vi "Straighten Up V2015.vi"(2 "stop":bool, 3 "10CM?":bool, 4 "Estimated Location":u16(ring) items=["Center Top", "Left Top", "Center Bottom", "Right Bottom", "Home", "Right mid", "Center Top 0", "Panting rowe"]) -> (0 "X Guess":i32, 1 "Y Guess":i32)   [LabVIEW 2014]
uses:
  <vilib>/userdefined/High Color/nirio_resource_hc.ctl
  <vilib>/FPGAPlugInAG/myRIO-1900/niLvFpga_Open_myRIO-1900.vi
  <vilib>/rvi/interface/common/dynamic/niFpgaDynamicAddResources.vi
  <vilib>/Utility/error.llb/Error Cluster From Error Code.vi
  <vilib>/rvi/errors/niLvFpgaAdjustHostInterfaceError.vi
  <vilib>/FPGAPlugInAG/Dynamic/niLvFpga_Close_Dynamic.vi
  <vilib>/rvi/interface/nirviOpenFPGA/nirviOpenFPGA.xnode
  FPGA Bitfiles/MITe2015_FPGATarget_FPGA-1900MotorAu_fQqeE40Xepw.lvbitx
  FPGA/FPGA-1900 Motor Automation Test.vi
  <vilib>/rvi/interface/nirviReadWriteControl/nirviReadWriteControl.xnode
  <vilib>/rvi/interface/nirviCloseFPGA/nirviCloseFPGA.xnode
  <vilib>/rvi/interface/Simulation/niFpgaSimulationCallBeginRW.vi
  NiFpgaLv.dll
panel:
  out "error out":errorcluster
  out "Center Right AVG":dbl
  out "Center Left AVG":dbl
  in  "Accuracy":dbl=0.3 format="%#_13g"
  out "STOP":bool
  out "Difrence":dbl
  out "F Left AVG":dbl
  out "F Right AVG":dbl
  out "Centre Right Dist (cm)":fxp<+,24,16>
  out "Centre Left Dist (cm)":fxp<+,24,16>
  out "Front Right Dist (cm)":fxp<+,24,16>
  out "Front Left Dist (cm)":fxp<+,24,16>
  in  "resource name":T1="RIO0"
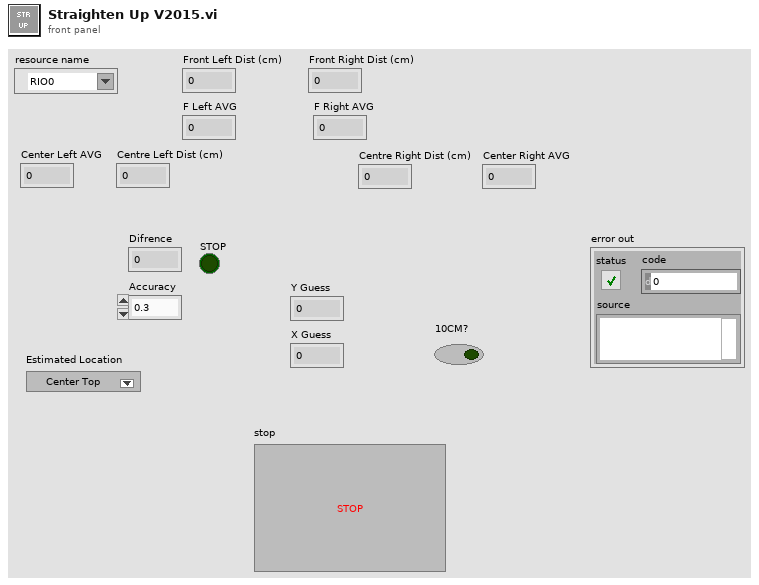
[diagram p1: front panel]
types:
  T1 = typedef "nirio_resource_hc.ctl" = tag
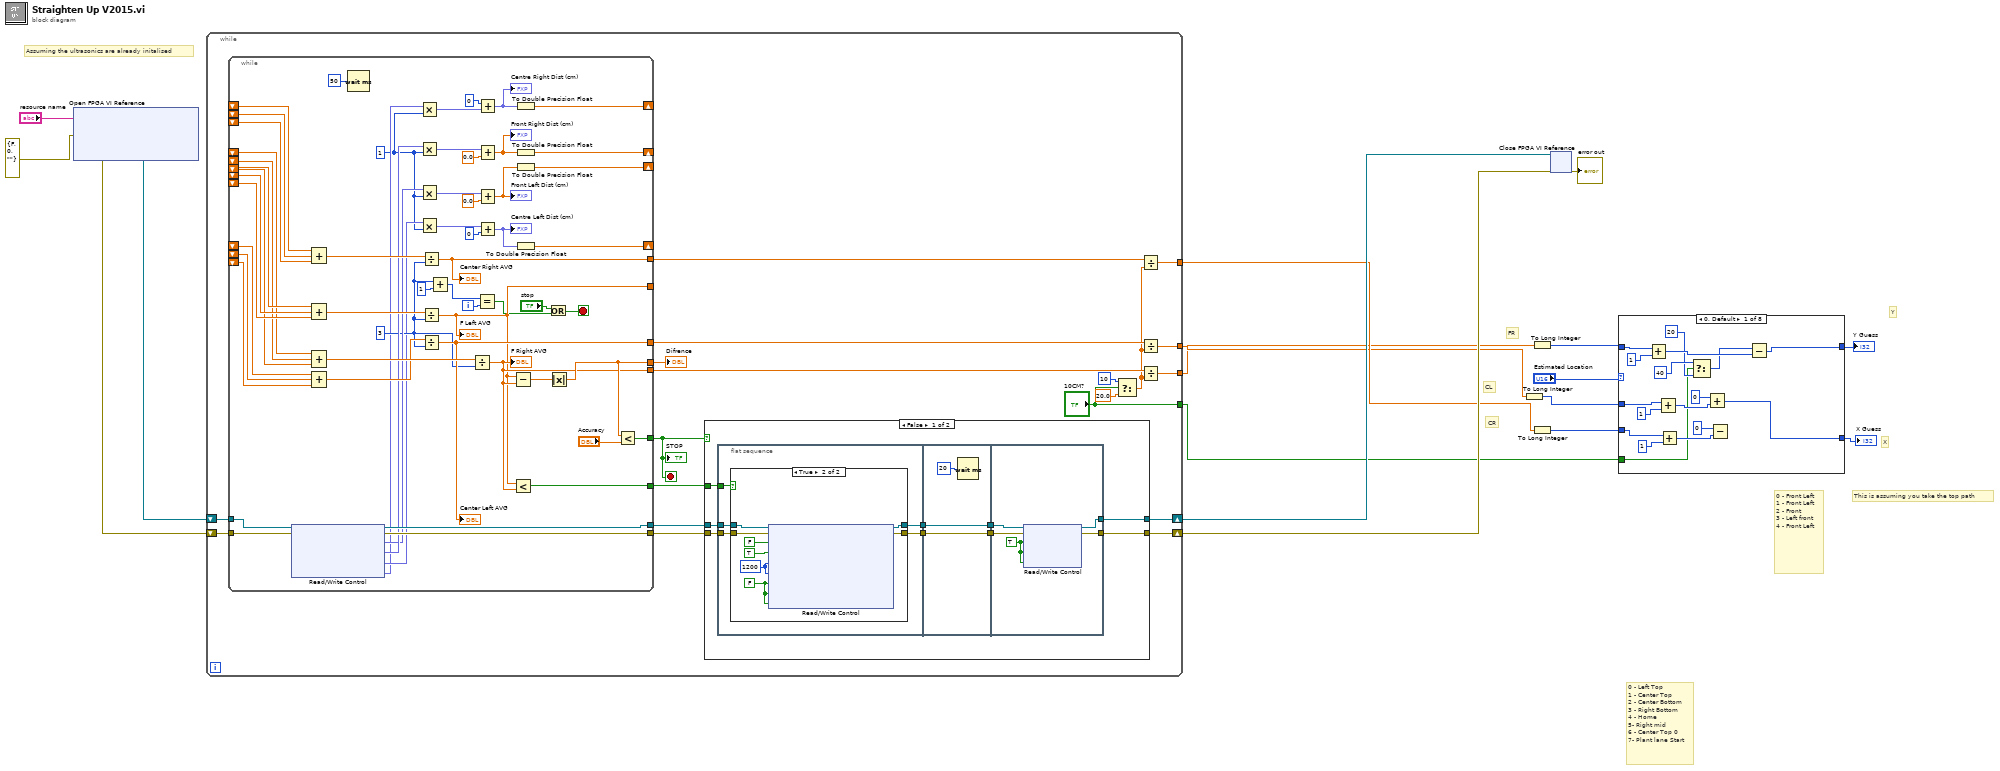
[diagram p0: block diagram]
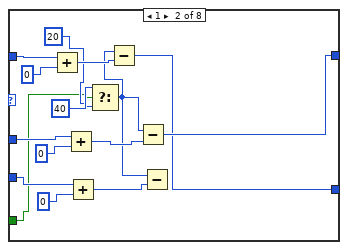
[diagram p2: hidden frame]
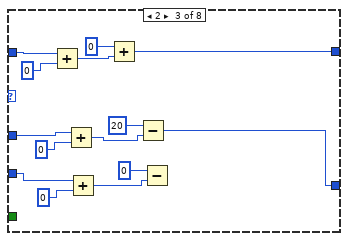
[diagram p3: hidden frame]
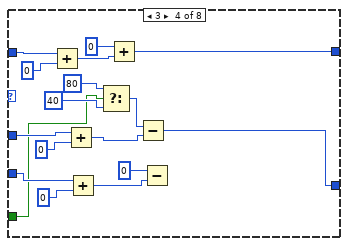
[diagram p4: hidden frame]
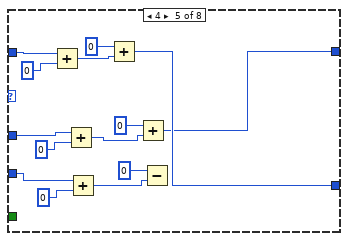
[diagram p5: hidden frame]
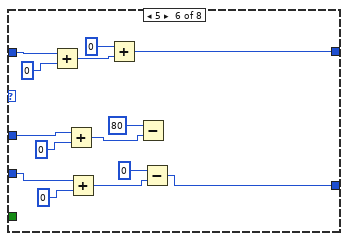
[diagram p6: hidden frame]
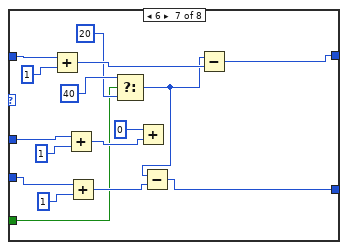
[diagram p7: hidden frame]
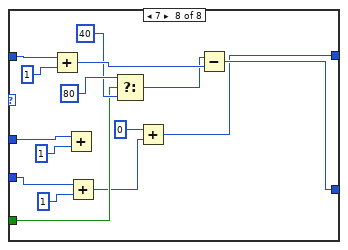
[diagram p8: hidden frame]
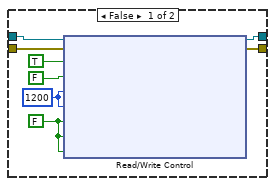
[diagram p9: hidden frame]
diagram:
  # "CR"
  # "CL"
  # "FR"
  # "X"
  # "Y"
  # "This is assuming you take the top path"
  # "0 - Front Left\n1 - Front Left\n2 - Front\n3 - Left front\n4 - Front Left"
  # "0 - Left Top\n1 - Center Top\n2 - Center Bottom\n3 - Right Bottom\n4 - Home\n5- Right mid\n6 - Center Top 0\n7- Plant lane Start"
  # "Assuming the ultrasonics are already initalised"
  n1 = xnode "Open FPGA VI Reference"("error in"=errorcluster {"status"=FALSE, "code"=0, "source"=""}, "resource name"="resource name") -> ("FPGA VI Reference Out"=w13:refnum<k20>, "error out"=w12:errorcluster)
  n2 = while {
    shift-right: [w33] -> w15
    shift-left: w13 -> [w28]
    shift-right: [w32] -> w14
    shift-left: w12 -> [w29]
    tunnel: [w23] -> w6
    tunnel: [w26] -> w7
    tunnel: [w25] -> w10
    tunnel: ["10CM?"] -> w2
    stop <- w30 stop-if-true
    n3 = while {
      tunnel: w28 -> [w133]
      tunnel: w29 -> [w132]
      tunnel: [w131] -> w35
      tunnel: [w130] -> w34
      shift-right: [w115] -> _
      shift-left: _ -> [w129]
      shift-right: [w113] -> _
      shift-left: _ -> [w126]
      shift-left: _ -> [w128]
      shift-left: _ -> [w127]
      shift-left: _ -> [w125]
      shift-left: _ -> [w124]
      tunnel: [w112] -> w36
      tunnel: [w109] -> w30
      tunnel: [w108] -> w31
      shift-right: [w104] -> _
      shift-left: _ -> [w101]
      shift-right: [w105] -> _
      shift-left: _ -> [w98]
      shift-left: _ -> [w100]
      shift-left: _ -> [w99]
      shift-left: _ -> [w97]
      shift-left: _ -> [w96]
      tunnel: [w93] -> w27
      tunnel: [w81] -> w18
      tunnel: [w92] -> w24
      tunnel: [w80] -> _
      i -> [w121]
      stop <- w77 stop-if-true
      w84 = 1 ("y")
      w87 = 3 ("y")
      n4 = xnode "Read/Write Control"("FPGA VI Reference In"=w133, "error in"=w132) -> ("FPGA VI Reference Out"=w131:refnum<k20>, "error out"=w130:errorcluster, "Front Left Dist (cm)"=w89:fxp<+,24,16>, "Front Right Dist (cm)"=w91:fxp<+,24,16>, "Centre Left Dist (cm)"=w86:fxp<+,24,16>, "Centre Right Dist (cm)"=w85:fxp<+,24,16>)
      n5 = Compound Arithmetic op=ADD(w98, w97, w96) -> (w94:dbl)
      n6 = Compound Arithmetic op=ADD(w129, w128, w127) -> (w123:dbl)
      n7 = Compound Arithmetic op=ADD(w126, w125, w124) -> (w122:dbl)
      n8 = Compound Arithmetic op=ADD(w101, w100, w99) -> (w95:dbl)
      n9 = Wait (ms)(milliseconds to wait=u32 50 ("millisecond multiple")) -> ()  [unwired: 1 out]
      n10 = Multiply(x=w85, y=w84) -> (x*y=w82:fxp<+/-,56,48>)
      n11 = Multiply(x=w91, y=w84) -> (x*y=w90:fxp<+/-,56,48>)
      n12 = Multiply(x=w89, y=w84) -> (x*y=w88:fxp<+/-,56,48>)
      n13 = Multiply(x=w86, y=w84) -> (x*y=w83:fxp<+/-,56,48>)
      n14 = Divide(x=w94, y=w87) -> (x/y=w81:dbl)
      "Center Right AVG" <- w81
      n15 = Divide(x=w123, y=w87) -> (x/y=w80:dbl)
      "F Left AVG" <- w80
      n16 = Divide(x=w95, y=w87) -> (x/y=w93:dbl)
      "Center Left AVG" <- w93
      n17 = Add(x=w87, y=1) -> (x+y=w119:i32)
      n18 = Divide(x=w122, y=w87) -> (x/y=w92:dbl)
      "F Right AVG" <- w92
      n19 = Equal?(x=w119, y=w121) -> (x = y?=w78:bool)
      n20 = Add(x=0, y=w82) -> (x+y=w102:fxp<+/-,57,49>)
      "Centre Right Dist (cm)" <- w102
      n21 = Add(x=w90, y=0.0 ("x")) -> (x+y=w114:dbl)
      "Front Right Dist (cm)" <- w114
      n22 = Add(x=w88, y=0.0 ("x")) -> (x+y=w116:dbl)
      "Front Left Dist (cm)" <- w116
      n23 = Add(x=w83, y=0 ("x")) -> (x+y=w103:fxp<+/-,57,49>)
      "Centre Left Dist (cm)" <- w103
      n24 = Subtract(x=w80, y=w92) -> (x-y=w111:dbl)
      n25 = Less?(x=w80, y=w92) -> (x < y?=w112:bool)
      n26 = To Double Precision Float(number=w102) -> (double precision float=w105:dbl)
      n27 = To Double Precision Float(number=w114) -> (double precision float=w113:dbl)
      n28 = To Double Precision Float(number=w116) -> (double precision float=w115:dbl)
      n29 = To Double Precision Float(number=w103) -> (double precision float=w104:dbl)
      n30 = Or(x="stop", y=w78) -> (x .or. y?=w77:bool)
      n31 = Absolute Value(x=w111) -> (abs(x)=w108:dbl)
      n32 = Less?(x=w108, y="Accuracy") -> (x < y?=w109:bool)
    }
    "Difrence" <- w31
    "STOP" <- w30
    n33 = case shown="False" w30 {
      tunnel: w36 -> [w41 _]
      tunnel: w35 -> [w40 w76]
      tunnel: w34 -> [w39 w75]
      tunnel: [w38 w76] -> w33
      tunnel: [w37 w75] -> w32
      frame False {
        n34 = flat-sequence {
          tunnel: w41 -> [w50]
          tunnel: w40 -> [w49]
          tunnel: w39 -> [w48]
          tunnel: [w47] -> w45
          tunnel: [w46] -> w44
          tunnel: w45 -> [w67]
          tunnel: [w68] -> w43
          tunnel: w44 -> [w68]
          tunnel: [w67] -> w42
          tunnel: w43 -> [w73]
          tunnel: w42 -> [w74]
          tunnel: [w72] -> w38
          tunnel: [w71] -> w37
          frame #0 {
            n35 = case shown="True" w50 {
              tunnel: w49 -> [w58 w66]
              tunnel: w48 -> [w57 w65]
              tunnel: [w56 w64] -> w47
              tunnel: [w55 w63] -> w46
              frame False {
                w53 = u32 1200 ("Right motor pulse width (uSec)")
                w51 = FALSE ("Right Motor")
                n36 = xnode "Read/Write Control"("FPGA VI Reference In"=w58, "error in"=w57, "Left Motor"=TRUE ("Right Motor"), "Right Motor"=FALSE, "Left motor pulse width (uSec)"=w53, "Right motor pulse width (uSec)"=w53, "Stop Left"=w51, "Stop Right"=w51, "Stop motors"=w51) -> ("FPGA VI Reference Out"=w56:refnum<k20>, "error out"=w55:errorcluster)
              }
              frame True {
                w61 = u32 1200 ("Right motor pulse width (uSec)")
                w59 = FALSE ("Right Motor")
                n37 = xnode "Read/Write Control"("FPGA VI Reference In"=w66, "error in"=w65, "Left Motor"=FALSE ("Right Motor"), "Right Motor"=TRUE, "Left motor pulse width (uSec)"=w61, "Right motor pulse width (uSec)"=w61, "Stop Left"=w59, "Stop Right"=w59, "Stop motors"=w59) -> ("FPGA VI Reference Out"=w64:refnum<k20>, "error out"=w63:errorcluster)
              }
            }
          }
          frame #1 {
            n38 = Wait (ms)(milliseconds to wait=20) -> ()  [unwired: 1 out]
          }
          frame #2 {
            w70 = TRUE ("Right Motor")
            n39 = xnode "Read/Write Control"("FPGA VI Reference In"=w74, "error in"=w73, "Stop Left"=w70, "Stop Right"=w70, "Stop motors"=w70) -> ("FPGA VI Reference Out"=w72:refnum<k20>, "error out"=w71:errorcluster)
          }
        }
      }
      frame True {
      }
    }
    n40 = Select(t=10, s="10CM?", f=20.0 ("y")) -> (s? t:f=w20:dbl)
    n41 = Divide(x=w18, y=w20) -> (x/y=w25:dbl)
    n42 = Divide(x=w27, y=w20) -> (x/y=w26:dbl)
    n43 = Divide(x=w24, y=w20) -> (x/y=w23:dbl)
  }
  n44 = To Long Integer(number=w7) -> (32bit integer=w8:i32)
  n45 = To Long Integer(number=w6) -> (32bit integer=w5:i32)
  n46 = To Long Integer(number=w10) -> (32bit integer=w9:i32)
  n47 = xnode "Close FPGA VI Reference"("FPGA VI Reference In"=w15, "error in"=w14) -> ("error out"=→"error out":errorcluster)
  n48 = case shown="0, Default" "Estimated Location" {
    tunnel: w8 -> [w144 w161 w172 w190 w203 w217 w235 w250]
    tunnel: w5 -> [w149 w166 w177 w195 w208 w222 w240 w255]
    tunnel: w9 -> [w145 w162 w173 w191 w204 w218 w236 w251]
    tunnel: [w135 w152 w167 w185 w199 w212 w226 w244] -> w4
    tunnel: [w136 w153 w168 w186 w198 w213 w227 w243] -> w3
    tunnel: w2 -> [w137 w155 _ w182 _ _ w229 w246]
    frame 0, Default {
      n49 = Add(x=w149, y=1 ("x")) -> (x+y=w143:i32)
      n50 = Add(x=w144, y=1 ("x")) -> (x+y=w142:i32)
      n51 = Add(x=w145, y=1 ("x")) -> (x+y=w141:i32)
      n52 = Select(t=40 ("x"), s=w137, f=20 ("x")) -> (s? t:f=w138:i32)
      n53 = Add(x=0, y=w142) -> (x+y=w135:i32)
      n54 = Subtract(x=0, y=w141) -> ()  [unwired: 1 out]
      n55 = Subtract(x=w138, y=w143) -> (x-y=w136:i32)
    }
    frame 1 {
      n56 = Add(x=w166, y=0 ("x")) -> (x+y=w160:i32)
      n57 = Add(x=w161, y=0 ("x")) -> (x+y=w159:i32)
      n58 = Add(x=w162, y=0 ("x")) -> (x+y=w158:i32)
      n59 = Select(t=40 ("x"), s=w155, f=20 ("x")) -> (s? t:f=w154:i32)
      n60 = Subtract(x=w154, y=w160) -> (x-y=w152:i32)
      n61 = Subtract(x=w154, y=w159) -> (x-y=w153:i32)
      n62 = Subtract(x=w154, y=w158) -> ()  [unwired: 1 out]
    }
    frame 2 {
      n63 = Add(x=w177, y=0 ("x")) -> (x+y=w171:i32)
      n64 = Add(x=w172, y=0 ("x")) -> (x+y=w170:i32)
      n65 = Add(x=w173, y=0 ("x")) -> (x+y=w169:i32)
      n66 = Add(x=0, y=w171) -> (x+y=w168:i32)
      n67 = Subtract(x=20, y=w170) -> (x-y=w167:i32)
      n68 = Subtract(x=0, y=w169) -> ()  [unwired: 1 out]
    }
    frame 3 {
      n69 = Add(x=w195, y=0 ("x")) -> (x+y=w189:i32)
      n70 = Add(x=w190, y=0 ("x")) -> (x+y=w188:i32)
      n71 = Add(x=w191, y=0 ("x")) -> (x+y=w187:i32)
      n72 = Select(t=80 ("x"), s=w182, f=40 ("x")) -> (s? t:f=w181:i32)
      n73 = Add(x=0, y=w189) -> (x+y=w186:i32)
      n74 = Subtract(x=w181, y=w188) -> (x-y=w185:i32)
      n75 = Subtract(x=0, y=w187) -> ()  [unwired: 1 out]
    }
    frame 4 {
      n76 = Add(x=w208, y=0 ("x")) -> (x+y=w202:i32)
      n77 = Add(x=w203, y=0 ("x")) -> (x+y=w201:i32)
      n78 = Add(x=w204, y=0 ("x")) -> (x+y=w200:i32)
      n79 = Add(x=0, y=w202) -> (x+y=w199:i32)
      n80 = Add(x=0, y=w201) -> (x+y=w198:i32)
      n81 = Subtract(x=0, y=w200) -> ()  [unwired: 1 out]
    }
    frame 5 {
      n82 = Add(x=w222, y=0 ("x")) -> (x+y=w216:i32)
      n83 = Add(x=w217, y=0 ("x")) -> (x+y=w215:i32)
      n84 = Add(x=w218, y=0 ("x")) -> (x+y=w214:i32)
      n85 = Add(x=0, y=w216) -> (x+y=w213:i32)
      n86 = Subtract(x=80, y=w215) -> ()  [unwired: 1 out]
      n87 = Subtract(x=0, y=w214) -> (x-y=w212:i32)
    }
    frame 6 {
      n88 = Add(x=w240, y=1 ("x")) -> (x+y=w234:i32)
      n89 = Add(x=w235, y=1 ("x")) -> (x+y=w233:i32)
      n90 = Add(x=w236, y=1 ("x")) -> (x+y=w232:i32)
      n91 = Select(t=40 ("x"), s=w229, f=20 ("x")) -> (s? t:f=w228:i32)
      n92 = Add(x=0, y=w233) -> ()  [unwired: 1 out]
      n93 = Subtract(x=w228, y=w232) -> (x-y=w226:i32)
      n94 = Subtract(x=w228, y=w234) -> (x-y=w227:i32)
    }
    frame 7 {
      n95 = Add(x=w255, y=1 ("x")) -> (x+y=w249:i32)
      n96 = Add(x=w250, y=1 ("x")) -> ()  [unwired: 1 out]
      n97 = Add(x=w251, y=1 ("x")) -> (x+y=w242:i32)
      n98 = Select(t=80 ("x"), s=w246, f=40 ("x")) -> (s? t:f=w245:i32)
      n99 = Add(x=0, y=w242) -> (x+y=w243:i32)
      n100 = Subtract(x=w245, y=w249) -> (x-y=w244:i32)
    }
  }
  "X Guess" <- w4
  "Y Guess" <- w3
